vi "Abbreviate_string.vi"(4 "Input String":string, 5 "Max String Length":i32=50) -> (0 "finalLength":i32, 1 "Output String":string, 2 "needMoreWidth":bool)   [LabVIEW 2021]
panel:
  out "audit":string[](array[string])
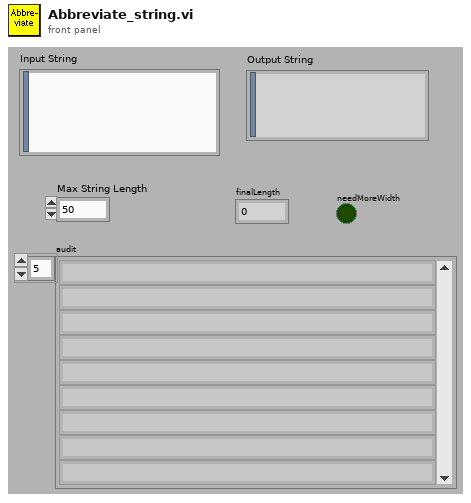
[diagram p1: front panel]
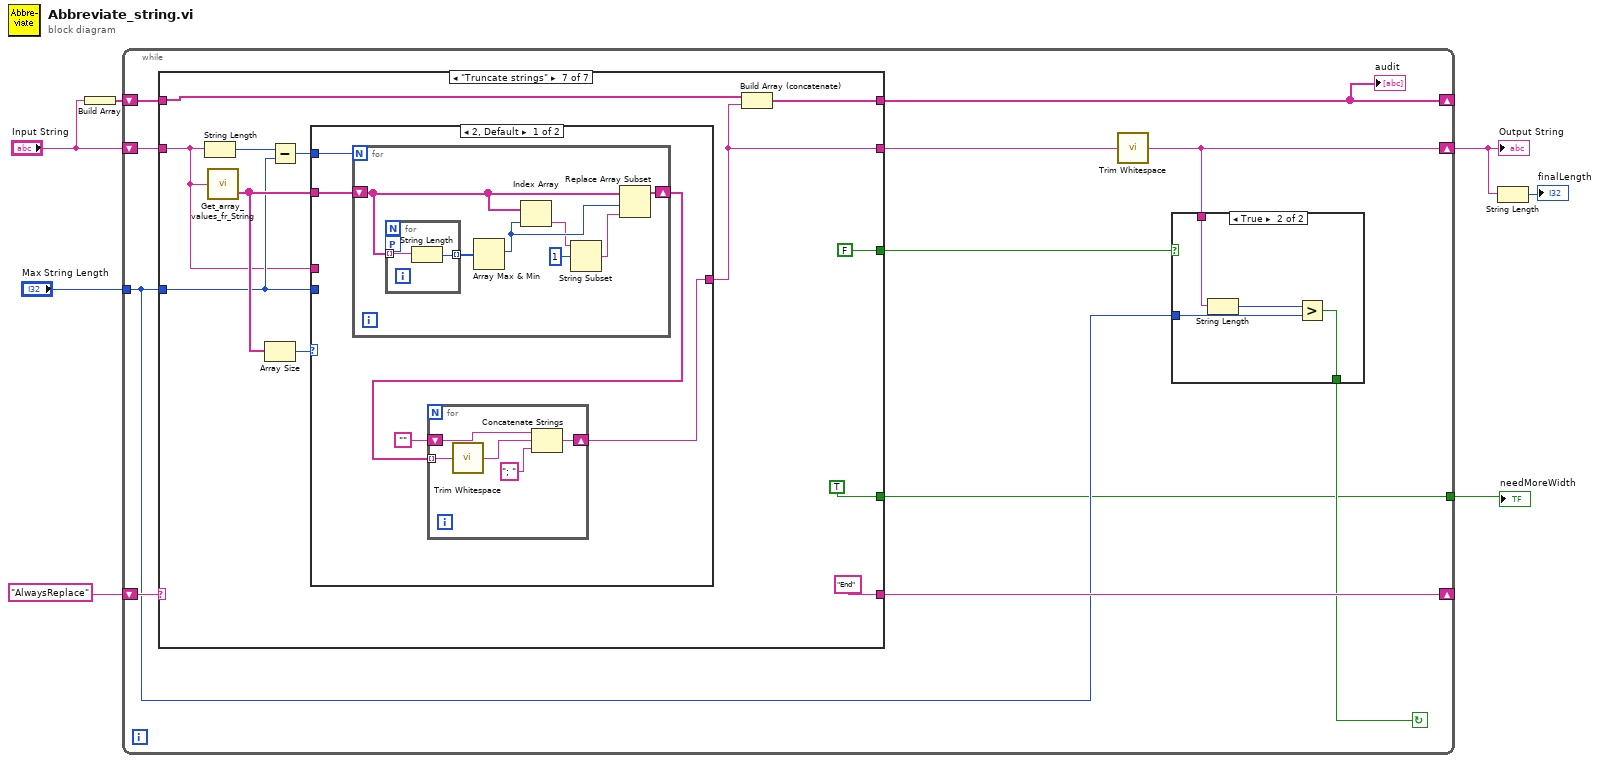
[diagram p0: block diagram]
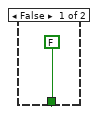
[diagram p2: hidden frame]
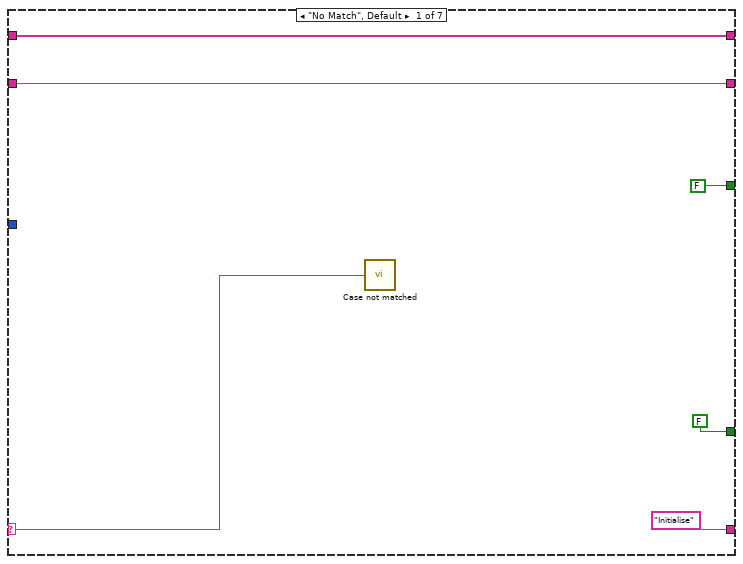
[diagram p3: hidden frame]
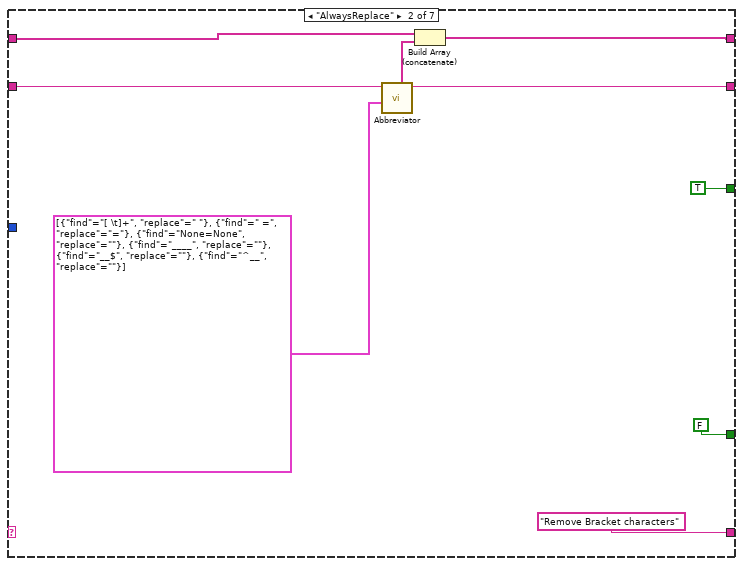
[diagram p4: hidden frame]
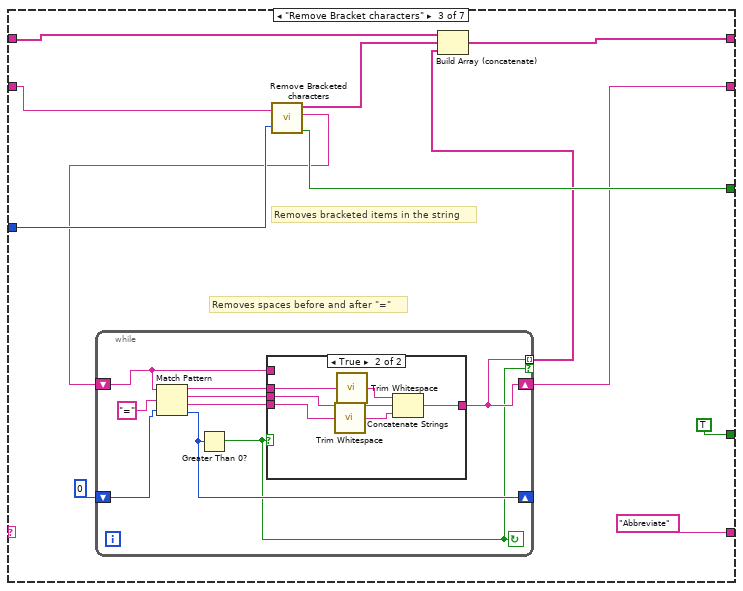
[diagram p5: hidden frame]
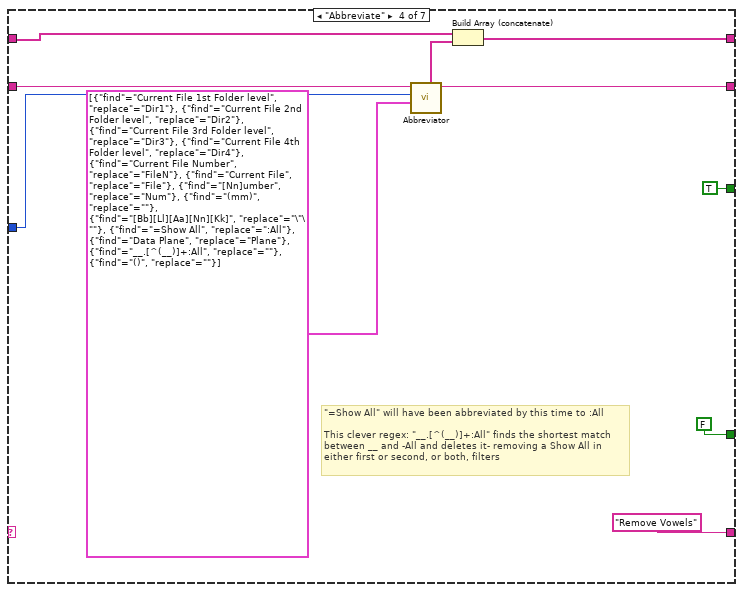
[diagram p7: hidden frame]
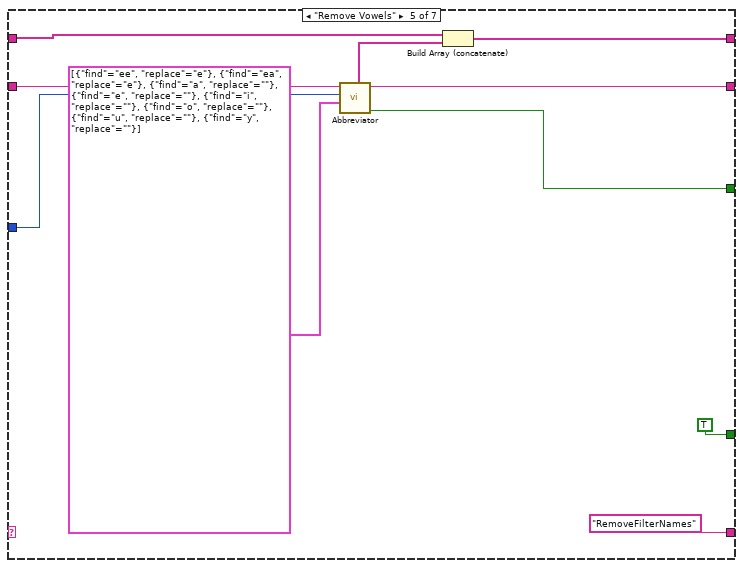
[diagram p8: hidden frame]
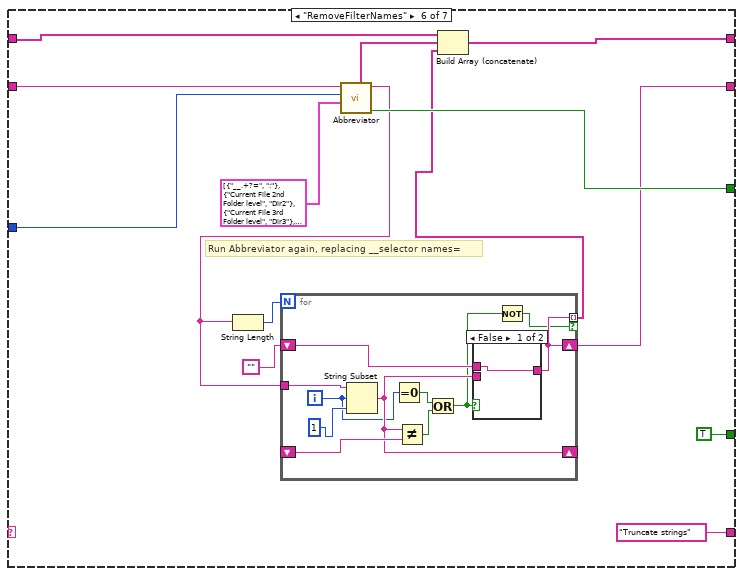
[diagram p9: hidden frame]
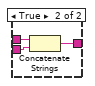
[diagram p10: hidden frame]
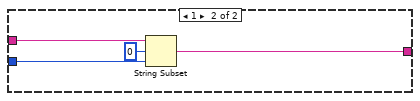
[diagram p11: hidden frame]
diagram:
  n1 = Build Array("Input String") -> (w1:string[])
  n2 = while {
    shift-left: "AlwaysReplace" -> [w17]
    shift-right: [w18] -> _
    shift-right: [w10] -> w4
    shift-left: "Input String" -> [w16]
    tunnel: "Max String Length" -> [w15]
    tunnel: [w11] -> w3
    shift-right: [w8] -> _
    shift-left: w1 -> [w9]
    stop <- w13 continue-if-true
    n3 = case shown="\"Truncate strings\"" w17 {
      selector: w17 -> [w26 _ _ _ _ _ _]
      tunnel: [FALSE TRUE w43 TRUE w82 w96 FALSE] -> w14
      tunnel: ["Initialise" "Remove Bracket characters" "Abbreviate" "Remove Vowels" "RemoveFilterNames" "Truncate strings" "End"] -> w18
      tunnel: w16 -> [w27 w36 w46 w74 w84 w98 w120]
      tunnel: w15 -> [_ _ w44 w71 w83 w97 w121]
      tunnel: [w27 w35 w41 w72 w77 w88 w116] -> w12
      tunnel: [FALSE FALSE TRUE FALSE TRUE TRUE TRUE] -> w11
      tunnel: [w24 w30 w48 w68 w80 w94 w118] -> w8
      tunnel: w9 -> [w24 w32 w47 w67 w78 w93 w117]
      frame "No Match", Default {
        n4 = call "Case not matched.vi"("Case Name not Matched"=w26) -> ()
      }
      frame "AlwaysReplace" {
        n5 = call "Abbreviator.vi"("replaceArray"=cluster{"find":string, "replace":string}[] [{"find"="[ \t]+", "replace"=" "}, {"find"=" =", "replace"="="}, {"find"="None=None", "replace"=""}, {"find"="____", "replace"=""}, {"find"="__$", "replace"=""}, {"find"="^__", "replace"=""}], "longStringIn"=w36) -> ("shortStringOut"=w35:string, "audit"=w31:string[])  [unwired: 6 in, 2 out]
        n6 = Build Array (concatenate)(w32, w31) -> (w30:string[])
      }
      frame "Remove Bracket characters" {
        # "Removes spaces before and after \"=\""
        # "Removes bracketed items in the string"
        n7 = call "Remove Bracketed characters.vi"("Input String"=w46, "Max String Length (0)"=w44) -> ("audit"=w45:string[], "Output String"=w42:string, "stillTooLong"=w43:bool)  [unwired: 1 out]
        n8 = while {
          shift-right: [w52] -> w41
          shift-left: w42 -> [w55]
          shift-right: [w54] -> _
          shift-left: 0 ("offset past match") -> [w53]
          tunnel: [w52] -> w40 mode=indexing if=w51
          stop <- w51 continue-if-true
          n9 = Match Pattern(string=w55, regular expression="=", offset (0)=w53) -> (before substring=w58:string, match substring=w56:string, after substring=w57:string, offset past match=w54:i32)
          n10 = Greater Than 0?(x=w54) -> (x > 0?=w51:bool)
          n11 = case shown="True" w51 {
            tunnel: w58 -> [_ w66]
            tunnel: w57 -> [_ w65]
            tunnel: w56 -> [_ w63]
            tunnel: [w60 w61] -> w52
            tunnel: w55 -> [w60 _]
            frame False {
            }
            frame True {
              n12 = call <vilib>:"Trim Whitespace.vi"("string"=w65) -> ("trimmed string"=w62:string)  [unwired: 1 in]
              n13 = call <vilib>:"Trim Whitespace.vi"("string"=w66) -> ("trimmed string"=w64:string)  [unwired: 1 in]
              n14 = Concatenate Strings(w64, w63, w62) -> (w61:string)
            }
          }
        }
        n15 = Build Array (concatenate)(w47, w45, w40) -> (w48:string[])
      }
      frame "Abbreviate" {
        # "\"=Show All\" will have been abbreviated by this time to :All\n\nThis clever regex: \"__.[^(__)]+:All\" finds the shortest match between __ and -All and deletes it- removing a Show All in either first or second, or both, filters"
        n16 = call "Abbreviator.vi"("replaceArray"=cluster{"find":string, "replace":string}[] [{"find"="Current File 1st Folder level", "replace"="Dir1"}, {"find"="Current File 2nd Folder level", "replace"="Dir2"}, {"find"="Current File 3rd Folder level", "replace"="Dir3"}, {"find"="Current File 4th Folder level", "replace"="Dir4"}, {"find"="Current File Number", "replace"="FileN"}, {"find"="Current File", "replace"="File"}, {"find"="[Nn]umber", "replace"="Num"}, {"find"="(mm)", "replace"=""}, {"find"="[Bb][Ll][Aa][Nn][Kk]", "replace"="\"\""}, {"find"="=Show All", "replace"=":All"}, {"find"="Data Plane", "replace"="Plane"}, {"find"="__.[^(__)]+:All", "replace"=""}, {"find"="()", "replace"=""}], "Max String Length (0)"=w71, "longStringIn"=w74) -> ("shortStringOut"=w72:string, "audit"=w69:string[])  [unwired: 5 in, 2 out]
        n17 = Build Array (concatenate)(w67, w69) -> (w68:string[])
      }
      frame "Remove Vowels" {
        n18 = call "Abbreviator.vi"("replaceArray"=cluster{"find":string, "replace":string}[] [{"find"="ee", "replace"="e"}, {"find"="ea", "replace"="e"}, {"find"="a", "replace"=""}, {"find"="e", "replace"=""}, {"find"="i", "replace"=""}, {"find"="o", "replace"=""}, {"find"="u", "replace"=""}, {"find"="y", "replace"=""}], "Max String Length (0)"=w83, "longStringIn"=w84) -> ("stillTooLong"=w82:bool, "shortStringOut"=w77:string, "audit"=w79:string[])  [unwired: 5 in, 1 out]
        n19 = Build Array (concatenate)(w78, w79) -> (w80:string[])
      }
      frame "RemoveFilterNames" {
        # "Run Abbreviator again, replacing __selector names="
        n20 = call "Abbreviator.vi"("replaceArray"=cluster{"find":string, "replace":string}[] [{"find"="__.+?=", "replace"=":"}, {"find"="Current File 2nd Folder level", "replace"="Dir2"}, {"find"="Current File 3rd Folder level", "replace"="Dir3"}, {"find"="Current File 4th Folder level", "replace"="Dir4"}, {"find"="Current File Number", "replace"="FileN"}, {"find"="Current File", "replace"="File"}, {"find"="(mm)", "replace"=""}, {"find"="=Show All", "replace"=":All"}, {"find"="Data Plane", "replace"="Plane"}, {"find"="__.[^(__)]+:All", "replace"=""}, {"find"="__.+?=", "replace"=":"}], "Max String Length (0)"=w97, "longStringIn"=w98) -> ("stillTooLong"=w96:bool, "shortStringOut"=w89:string, "audit"=w92:string[])  [unwired: 5 in, 1 out]
        n21 = String Length(string=w89) -> (length=w91:i32)
        n22 = for {
          N: w91 -> [_]
          shift-right: [w108] -> _
          shift-left: _ -> [w110]
          shift-right: [w103] -> w88
          shift-left: "" -> [w109]
          tunnel: w89 -> [w104]
          tunnel: [w103] -> w87 mode=indexing if=w102
          i -> [w107]
          n23 = String Subset(string=w104, offset (0)=w107, length (rest)=1 ("length (rest)")) -> (substring=w108:string)
          n24 = Equal To 0?(x=w107) -> (x = 0?=w106:bool)
          n25 = Not Equal?(x=w108, y=w110) -> (x != y?=w105:bool)
          n26 = Or(x=w106, y=w105) -> (x .or. y?=w101:bool)
          n27 = case shown="False" w101 {
            tunnel: w109 -> [w112 w115]
            tunnel: [w112 w114] -> w103
            tunnel: w108 -> [_ w113]
            frame False {
            }
            frame True {
              n28 = Concatenate Strings(w115, w113) -> (w114:string)
            }
          }
          n29 = Not(x=w101) -> (.not. x?=w102:bool)
        }
        n30 = Build Array (concatenate)(w93, w92, w87) -> (w94:string[])
      }
      frame "Truncate strings" {
        n31 = String Length(string=w120) -> (length=w126:i32)
        n32 = call "Get_array_values_fr_String.vi"("String Value"=w120) -> ("String array"=w123:string[])  [unwired: 1 out]
        n33 = Array Size(array=w123) -> (size(s)=w122:i32)
        n34 = Subtract(x=w126, y=w121) -> (x-y=w125:i32)
        n35 = case shown="2, Default" w122 {
          tunnel: w125 -> [w132 _]
          tunnel: [w129 w147] -> w116
          tunnel: w123 -> [w128 _]
          tunnel: w121 -> [_ w150]
          tunnel: w120 -> [_ w148]
          frame 2, Default {
            n36 = for {
              N: w132 -> [_]
              shift-right: [w141] -> w131
              shift-left: w128 -> [w142]
              n37 = for {
                tunnel: w142 -> [w146] mode=indexing
                tunnel: [w145] -> w144 mode=indexing
                workers-P: _ -> [_]
                n38 = String Length(string=w146) -> (length=w145:i32)
              }
              n39 = Array Max & Min(array=w144) -> (max index (indices)=w143:i32)  [unwired: 3 out]
              n40 = Index Array(array=w142, index=w143) -> (element=w139:string)
              n41 = String Subset(string=w139, offset (0)=1) -> (substring=w138:string)  [unwired: 1 out]
              n42 = Replace Array Subset(array=w142, new element=w138, index=w143) -> (w141:string[])
            }
            n43 = for {
              shift-right: [w135] -> w129
              shift-left: "" -> [w137]
              tunnel: w131 -> [w134] mode=indexing
              n44 = call <vilib>:"Trim Whitespace.vi"("string"=w134) -> ("trimmed string"=w133:string)  [unwired: 1 in]
              n45 = Concatenate Strings(w137, w133, "; " ("string")) -> (w135:string)
            }
          }
          frame 1 {
            n46 = String Subset(string=w148, offset (0)=0, length (rest)=w150) -> (substring=w147:string)
          }
        }
        n47 = Build Array (concatenate)(w117, w116) -> (w118:string[])
      }
    }
    "audit" <- w8
    n48 = call <vilib>:"Trim Whitespace.vi"("string"=w12) -> ("trimmed string"=w10:string)  [unwired: 1 in]
    n49 = case shown="True" w14 {
      tunnel: w10 -> [_ w22]
      tunnel: w15 -> [_ w21]
      tunnel: [FALSE w20] -> w13
      frame False {
      }
      frame True {
        n50 = String Length(string=w22) -> (length=w23:i32)
        n51 = Greater?(x=w23, y=w21) -> (0:w20:bool)
      }
    }
  }
  "Output String" <- w4
  "needMoreWidth" <- w3
  n52 = String Length(string=w4) -> (length=→"finalLength":i32)
